vi "processData.vi"(8 "error in (no error)":errorcluster, 10 "model":refnum<class "Model.lvclass">, 11 "ControlledMotionState in":refnum<class "ControlledMotionState.lvclass">) -> (0 "error out":errorcluster, 2 "model 2":refnum<class "Model.lvclass">, 3 "ControlledMotionState out":refnum<class "ControlledMotionState.lvclass">)   [LabVIEW 2013, in "ControlledMotionState.lvclass"]
uses:
  ControlledMotionState.lvclass
  Model/Model/Model.lvclass
  EnabledState/EnabledState.lvclass
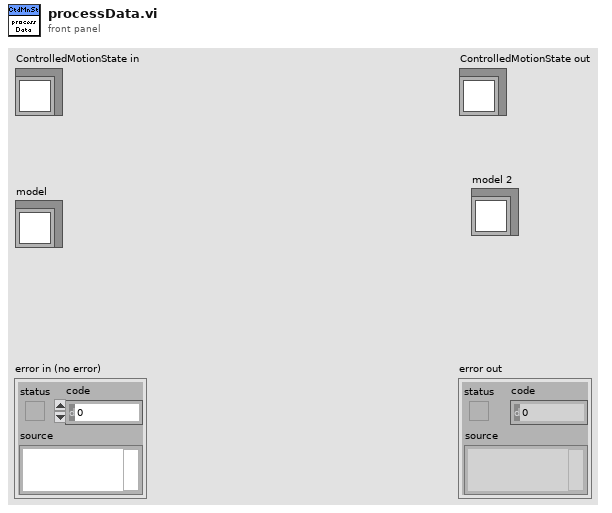
[diagram p1: front panel]
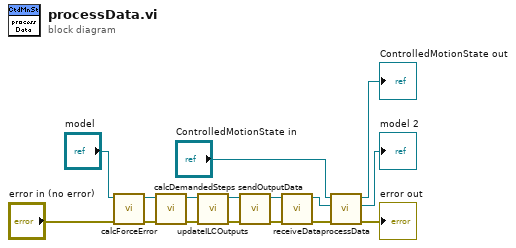
[diagram p0: block diagram]
diagram:
  n1 = call "calcForceError.vi"("error in (no error)"="error in (no error)", "Model in"="model") -> ("error out"=w9:errorcluster, "Model out"=w11:refnum<class "Model.lvclass">)  [unwired: 8 in]
  n2 = call "calcDemandedSteps.vi"("error in (no error)"=w9, "Model in"=w11) -> ("error out"=w6:errorcluster, "Model out"=w8:refnum<class "Model.lvclass">)  [unwired: 8 in]
  n3 = call "updateILCOutputs.vi"("error in (no error)"=w6, "Model in"=w8) -> ("error out"=w5:errorcluster, "Model out"=w7:refnum<class "Model.lvclass">)  [unwired: 8 in]
  n4 = call "sendOutputData.vi"("error in (no error)"=w5, "Model in"=w7) -> ("error out"=w2:errorcluster, "Model out"=w4:refnum<class "Model.lvclass">)  [unwired: 8 in]
  n5 = call "receiveData.vi"("error in (no error)"=w2, "Model in"=w4) -> ("error out"=w1:errorcluster, "Model out"=w3:refnum<class "Model.lvclass">)  [unwired: 8 in]
  n6 = call-parent "processData.vi"("error in (no error)"=w1, "model"=w3, "EnabledState in"="ControlledMotionState in") -> ("error out"=→"error out":errorcluster, "model 2"=→"model 2":refnum<class "Model.lvclass">, "EnabledState out"=→"ControlledMotionState out":refnum<class "ControlledMotionState.lvclass">)  [unwired: 6 in]
